vi "Item_Init.vi"(11 "Object":T1) -> ()   [LabVIEW 2020, in "FlexWorker_Provider.lvlib"]
uses:
  FlexWorker_Provider.lvlib
  <resource>/Framework/Providers/API/mxLvUpdateUI.ctl
  <resource>/Framework/Providers/API/mxLvOverlayState.ctl
  <resource>/Framework/Providers/API/ItemRef.ctl
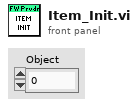
[diagram p1: front panel]
types:
  T1 = typedef "ItemRef.ctl" = u64
  T2 = typedef "mxLvOverlayState.ctl" = cluster{"Overlay Alias":string, "Active":bool}
  T3 = typedef "mxLvUpdateUI.ctl" = cluster{"Action":u32, "Optional param 1":string, "Optional param 2":i32, "Optional param 3":string}
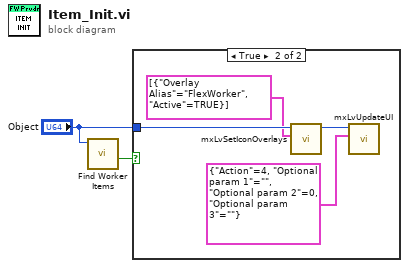
[diagram p0: block diagram]
diagram:
  n1 = call "Find Worker Items.vi"("Item Ref In"="Object") -> ("Is Worker?"=w1:bool)  [unwired: 8 in, 2 out]
  n2 = case shown="True" w1 {
    tunnel: "Object" -> [_ w4]
    frame False {
    }
    frame True {
      n3 = call <resource>:"mxLvSetIconOverlays.vi"("Overlay States"=T2[] [{"Overlay Alias"="FlexWorker", "Active"=TRUE}], "Item"=w4) -> ("Item"=w5:T1)  [unwired: 8 in, 1 out]
      n4 = call <resource>:"mxLvUpdateUI.vi"("Update UI Settings"=T3 {"Action"=4, "Optional param 1"="", "Optional param 2"=0, "Optional param 3"=""}, "Item"=w5) -> ()  [unwired: 8 in, 2 out]
    }
  }
